vi "DataGraph_MouseInit.vi"(7 "State":enum16{"Read", "Write"}(ring), 8 "error in (no error)":errorcluster, 10 "Coords":T2, 11 "Mass_Graph":refnum<vi>) -> (0 "error out":errorcluster, 2 "Point32":T2, 3 "reference out":refnum<vi>, 5 "Boundary":T1)   [LabVIEW 2018, in "DataGraphXControl.xctl"]
uses:
  DataGraphXControl.xctl
  <vilib>/Utility/miscctls.llb/LVPoint32TypeDef.ctl
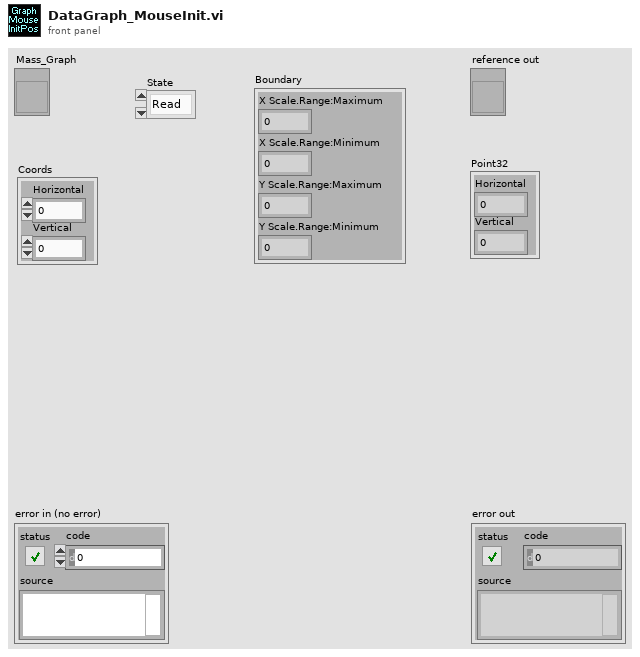
[diagram p1: front panel]
types:
  T1 = cluster{"X Scale.Range:Maximum":dbl, "X Scale.Range:Minimum":dbl, "Y Scale.Range:Maximum":dbl, "Y Scale.Range:Minimum":dbl}
  T2 = typedef "LVPoint32TypeDef.ctl" = cluster{"Horizontal":i32, "Vertical":i32}
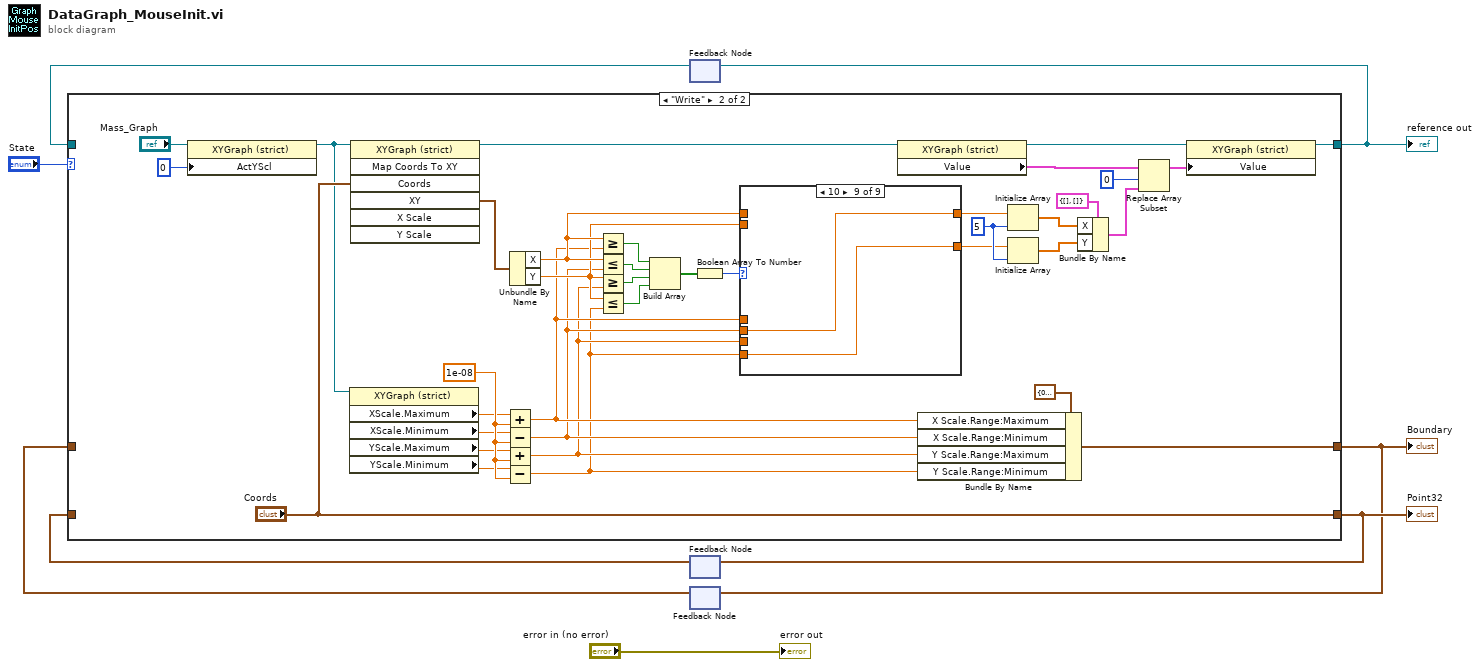
[diagram p0: block diagram]
diagram:
  n1 = feedback #1() -> (w3:refnum<vi>)  [unwired: 1 in]
  n2 = feedback #2() -> (w6:T2)  [unwired: 1 in]
  n3 = feedback #3() -> (w2:T1)  [unwired: 1 in]
  n4 = case shown="\"Write\"" "State" {
    tunnel: [w10 w36] -> w4
    tunnel: [w11 "Coords"] -> w5
    tunnel: w6 -> [w11 _]
    tunnel: w3 -> [w10 _]
    tunnel: w2 -> [w9 _]
    tunnel: [w9 w31] -> w1
    frame "Read", Default {
    }
    frame "Write" {
      w20 = 1e-08
      w41 = 5 ("dimension size")
      n5 = property class="XYGraph (strict)"(reference="Mass_Graph", "ActYScl"=0 ("Active Y Scale")) -> (reference out=w33:refnum<vi>)  [unwired: 1 in, 1 out]
      n6 = property class="XYGraph (strict)"(reference=w33) -> ("XScale.Maximum"=w16:dbl, "XScale.Minimum"=w19:dbl, "YScale.Maximum"=w18:dbl, "YScale.Minimum"=w17:dbl)  [unwired: 1 in, 2 out]
      n7 = invoke class="XYGraph (strict)" method="Map Coords To XY"(reference=w33, "Coords"="Coords") -> (reference out=w38:refnum<vi>, "XY"=w37:cluster{"X":dbl, "Y":dbl})  [unwired: 5 in, 5 out]
      n8 = Add(x=w16, y=w20) -> (x+y=w15:dbl)
      n9 = Subtract(x=w19, y=w20) -> (x-y=w14:dbl)
      n10 = Add(x=w18, y=w20) -> (x+y=w13:dbl)
      n11 = Subtract(x=w17, y=w20) -> (x-y=w12:dbl)
      n12 = Unbundle By Name(w37) -> ("X"=w24:dbl, "Y"=w23:dbl)
      n13 = Greater Or Equal?(x=w24, y=w15) -> (x >= y?=w30:bool)
      n14 = Less Or Equal?(x=w24, y=w14) -> (x <= y?=w29:bool)
      n15 = Greater Or Equal?(x=w23, y=w13) -> (x >= y?=w28:bool)
      n16 = Less Or Equal?(x=w23, y=w12) -> (x <= y?=w27:bool)
      n17 = Build Array(w30, w29, w28, w27) -> (w26:bool[])
      n18 = Boolean Array To Number(Boolean array=w26) -> (number=w25:u32)
      n19 = case shown="10" w25 {
        tunnel: w24 -> [w50 _ _ w56 _ _ w61 _ _]
        tunnel: w23 -> [w49 w51 w53 _ _ _ _ _ _]
        tunnel: w15 -> [_ w52 _ _ w57 _ _ w63 _]
        tunnel: w14 -> [_ _ w54 _ _ w60 _ _ w65]
        tunnel: w13 -> [_ _ _ w55 w58 w59 _ _ _]
        tunnel: w12 -> [_ _ _ _ _ _ w62 w64 w66]
        tunnel: [w50 w52 w54 w56 w57 w60 w61 w63 w65] -> w22
        tunnel: [w49 w51 w53 w55 w58 w59 w62 w64 w66] -> w21
        frame 0, Default {
        }
        frame 1 {
        }
        frame 2 {
        }
        frame 4 {
        }
        frame 5 {
        }
        frame 6 {
        }
        frame 8 {
        }
        frame 9 {
        }
        frame 10 {
        }
      }
      n20 = property class="XYGraph (strict)"(reference=w38) -> (reference out=w48:refnum<vi>, "Value"=w46:cluster{"X":dbl[], "Y":dbl[]}[])  [unwired: 1 in, 1 out]
      n21 = Bundle By Name(cluster=T1 {"X Scale.Range:Maximum"=0.0, "X Scale.Range:Minimum"=0.0, "Y Scale.Range:Maximum"=0.0, "Y Scale.Range:Minimum"=0.0} ("Boundary"), "X Scale.Range:Maximum"=w15, "X Scale.Range:Minimum"=w14, "Y Scale.Range:Maximum"=w13, "Y Scale.Range:Minimum"=w12) -> (w31:T1)
      n22 = Initialize Array(w22, w41) -> (w40:dbl[])
      n23 = Initialize Array(w21, w41) -> (w39:dbl[])
      n24 = Bundle By Name(cluster=cluster{"X":dbl[], "Y":dbl[]} {"X"=[], "Y"=[]} ("element"), "X"=w40, "Y"=w39) -> (w44:cluster{"X":dbl[], "Y":dbl[]})
      n25 = Replace Array Subset(array=w46, new element=w44, index=0) -> (w43:cluster{"X":dbl[], "Y":dbl[]}[])
      n26 = property class="XYGraph (strict)"(reference=w48, "Value"=w43) -> (reference out=w36:refnum<vi>)  [unwired: 1 in, 1 out]
    }
  }
  "reference out" <- w4
  "Point32" <- w5
  "Boundary" <- w1
  n27 = feedback-in #1(w4) -> ()
  n28 = feedback-in #2(w5) -> ()
  n29 = feedback-in #3(w1) -> ()
  "error out" <- "error in (no error)"
